vi "_PC_Pub_MS_EMA_Calc.vi"(6 "AVG Items in":u8, 7 "Init":bool, 8 "maxItems":u8=1, 9 "Y Data":sgl[](array[numeric]), 10 "EMACurrent in":sgl[](array[numeric]), 11 "EMAPrev in":sgl[](array[numeric])) -> (2 "EMACurrent out":sgl[](array[numeric]), 3 "EMAPrev out":sgl[](array[numeric]), 4 "AVG Items out":u8)   [LabVIEW 2018]
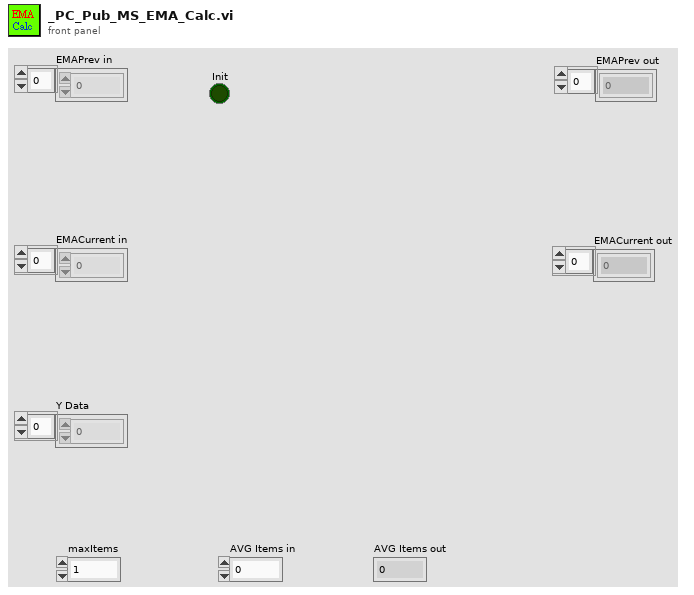
[diagram p1: front panel]
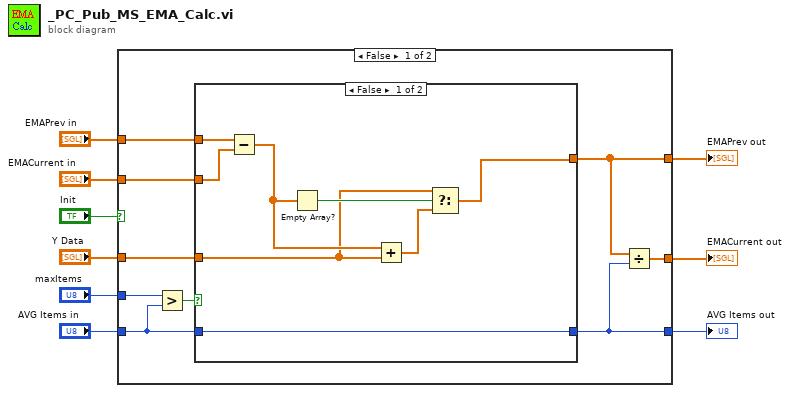
[diagram p0: block diagram]
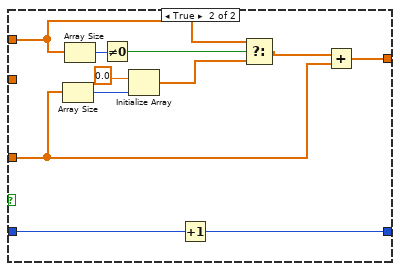
[diagram p2: hidden frame]
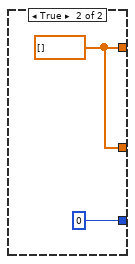
[diagram p3: hidden frame]
diagram:
  n1 = case shown="False" "Init" {
    tunnel: [w16 w38] -> w7
    tunnel: "AVG Items in" -> [w12 _]
    tunnel: [w13 u8 0 ("AVG Items in")] -> w8
    tunnel: "EMAPrev in" -> [w17 _]
    tunnel: [w15 w38] -> w6
    tunnel: "EMACurrent in" -> [w14 _]
    tunnel: "Y Data" -> [w11 _]
    tunnel: "maxItems" -> [w10 _]
    frame False {
      n2 = Greater?(x=w10, y=w12) -> (0:w18:bool)
      n3 = case shown="False" w18 {
        tunnel: w17 -> [w26 w30]
        tunnel: w11 -> [w20 w35]
        tunnel: [w19 w37] -> w16
        tunnel: w14 -> [w25 _]
        tunnel: [w24 w27] -> w13
        tunnel: w12 -> [w24 w28]
        frame False {
          n4 = Subtract(x=w26, y=w25) -> (x-y=w23:sgl[])
          n5 = Empty Array?(array=w23) -> (empty?=w22:bool)
          n6 = Add(x=w23, y=w20) -> (x+y=w21:sgl[])
          n7 = Select(t=w20, s=w22, f=w21) -> (s? t:f=w19:sgl[])
        }
        frame True {
          n8 = Array Size(array=w35) -> (size(s)=w33:i32)
          n9 = Array Size(array=w30) -> (size(s)=w36:i32)
          n10 = Not Equal To 0?(x=w36) -> (x != 0?=w34:bool)
          n11 = Initialize Array(sgl 0.0, w33) -> (w31:sgl[])
          n12 = Increment(x=w28) -> (x+1=w27:u8)
          n13 = Select(t=w30, s=w34, f=w31) -> (s? t:f=w29:sgl[])
          n14 = Add(x=w29, y=w35) -> (x+y=w37:sgl[])
        }
      }
      n15 = Divide(x=w16, y=w13) -> (x/y=w15:sgl[])
    }
    frame True {
      w38 = sgl[] []
    }
  }
  "EMACurrent out" <- w6
  "AVG Items out" <- w8
  "EMAPrev out" <- w7
